vi "Get Ingredients.vi"(8 "error in (no error)":errorcluster, 11 "Small Register Bank in":refnum<class "Small Register Bank.lvclass">) -> (0 "error out":errorcluster, 2 "Ingredients":T1[](array[typedef]), 3 "Small Register Bank out":refnum<class "Small Register Bank.lvclass">)   [LabVIEW 2020, in "Small Register Bank.lvclass"]
uses:
  Small Register Bank.lvclass
  Item/Ingredient.ctl
  Item/Item.lvclass
  Plastic Parts/Plastic Parts.lvclass
  C:/dev/IlluminatedG/lv-oopanel-gc-calc/Item/Item.lvclass
  Electronic Parts/Electronic Parts.lvclass
  Circuit Board/Circuit Board.lvclass
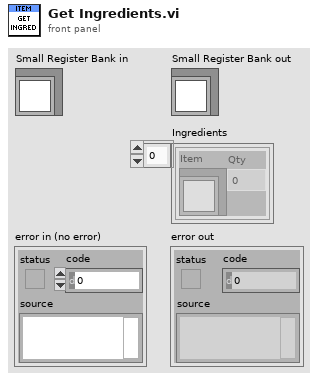
[diagram p1: front panel]
types:
  T1 = typedef "Item.lvclass/Ingredient.ctl" = cluster{"Item":refnum<class "Item.lvclass">, "Qty":dbl}
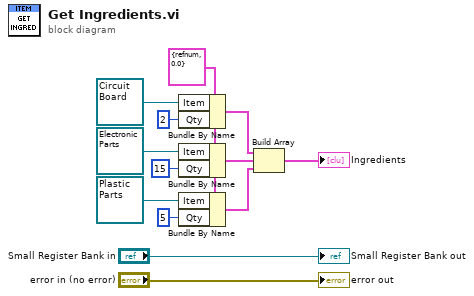
[diagram p0: block diagram]
diagram:
  w8 = T1 {"Item"=refnum, "Qty"=0.0} ("Ingredient")
  n1 = Bundle By Name(cluster=w8, "Item"=refnum<class "Circuit Board.lvclass"> refnum ("Circuit Board.lvclass"), "Qty"=2) -> (w5:T1)
  n2 = Bundle By Name(cluster=w8, "Item"=refnum<class "Electronic Parts.lvclass"> refnum ("Electronic Parts.lvclass"), "Qty"=15) -> (w7:T1)
  n3 = Bundle By Name(cluster=w8, "Item"=refnum<class "Plastic Parts.lvclass"> refnum ("Plastic Parts.lvclass"), "Qty"=5) -> (w6:T1)
  n4 = Build Array(w5, w7, w6) -> (→"Ingredients":T1[])
  "error out" <- "error in (no error)"
  "Small Register Bank out" <- "Small Register Bank in"
